vi "tpg361_set_unit.vi"() -> ()   [LabVIEW 2019]
panel:
  in  "SETTING UNIT":T1(ring)
  out "UNIT":string
  out "Overall Status":bool
  out "Acknowledgement Status":bool
  out "err_out":errorcluster
  out "tpg361_visa 2":refnum<visa-resource-name>
  in  "tpg361_b2r 2":u32
  in  "tpg361_delay 3":u32=500
  in  "tpg361_delay 2":u32=500
  in  "tpg361_b2r":u32
  in  "err_in":errorcluster
  in  "tpg361_delay":u32=500
  in  "tpg361_visa":refnum<visa-resource-name>
  # "VISA"
  # "DELAY"
  # "BYTE AT PORT"
  # "STATUS"
  # "ERROR"
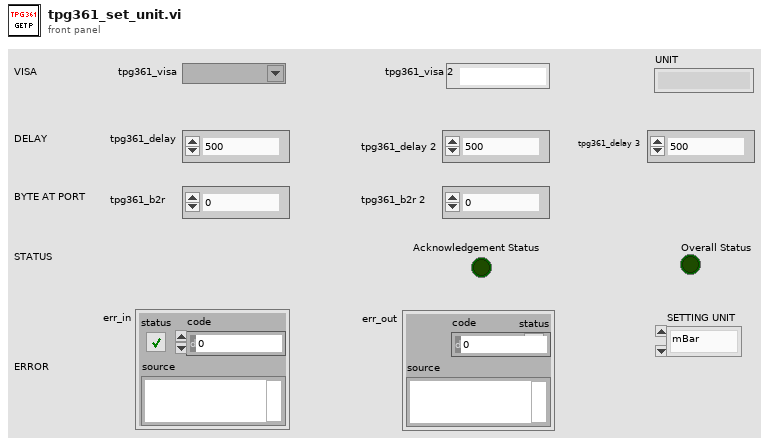
[diagram p1: front panel]
types:
  T1 = enum16{"mBar", "Torr", "Pascal", "micron", "hPascal", "Volt"}
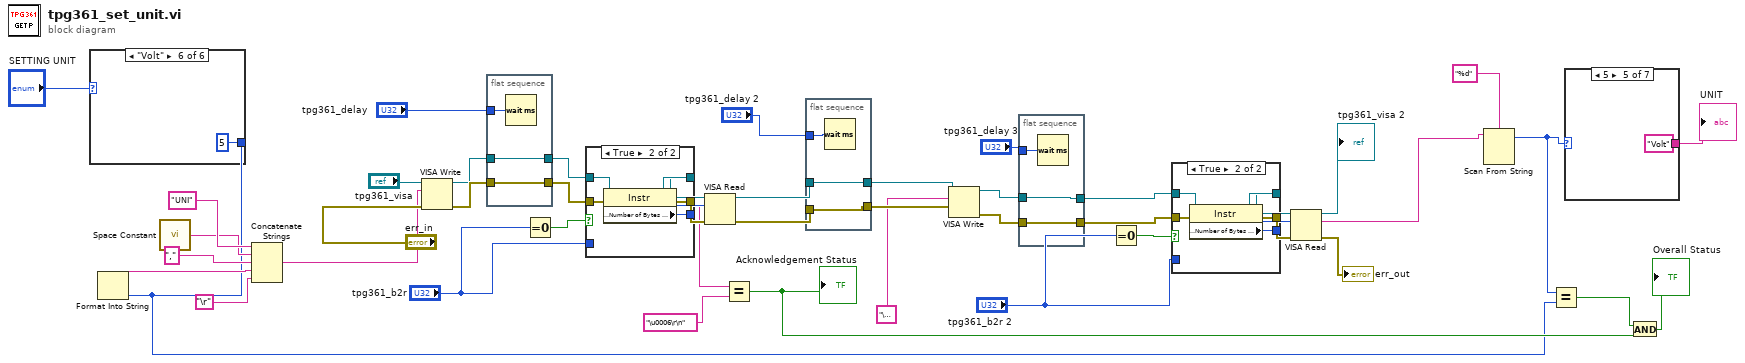
[diagram p0: block diagram]
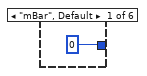
[diagram p2: hidden frame]
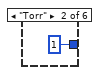
[diagram p3: hidden frame]
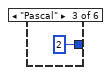
[diagram p4: hidden frame]
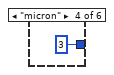
[diagram p5: hidden frame]
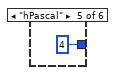
[diagram p6: hidden frame]
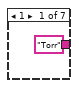
[diagram p7: hidden frame]
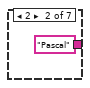
[diagram p8: hidden frame]
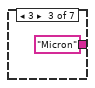
[diagram p9: hidden frame]
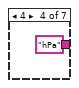
[diagram p10: hidden frame]
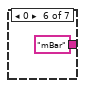
[diagram p11: hidden frame]
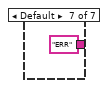
[diagram p12: hidden frame]
diagram:
  n1 = case shown="\"Volt\"" "SETTING UNIT" {
    tunnel: [0 1 2 3 4 5] -> w1
    frame "mBar", Default {
    }
    frame "Torr" {
    }
    frame "Pascal" {
    }
    frame "micron" {
    }
    frame "hPascal" {
    }
    frame "Volt" {
    }
  }
  n2 = Format Into String(w1) -> (resulting string=w6:string)  [unwired: 3 in, 1 out]
  n3 = call <vilib>:"Space Constant.vi"() -> ("String"=w8:string)
  n4 = Concatenate Strings("UNI" ("string"), w8, "," ("string"), w6, "\r") -> (w19:string)
  n5 = VISA Write(VISA resource name="tpg361_visa", write buffer=w19, error in (no error)="err_in") -> (VISA resource name out=w45:refnum<visa-resource-name>, error out=w47:errorcluster)  [unwired: 1 out]
  n6 = flat-sequence {
    tunnel: w47 -> [w55]
    tunnel: [w55] -> w46
    tunnel: w45 -> [w54]
    tunnel: [w54] -> w44
    tunnel: "tpg361_delay" -> [w56]
    frame #0 {
      n7 = Wait (ms)(milliseconds to wait=w56) -> ()  [unwired: 1 out]
    }
  }
  n8 = Equal To 0?(x="tpg361_b2r") -> (x = 0?=w40:bool)
  n9 = case shown="True" w40 {
    tunnel: w46 -> [w58 w64]
    tunnel: w44 -> [w59 w63]
    tunnel: [w59 w62] -> w38
    tunnel: [w58 w61] -> w37
    tunnel: [w57 w60] -> w36
    tunnel: "tpg361_b2r" -> [w57 _]
    frame False {
    }
    frame True {
      n10 = property class="Instr"(reference=w63, error in=w64) -> (reference out=w62:refnum<visa-resource-name>, error out=w61:errorcluster, "Serial Settings:Number of Bytes at Serial Port"=w60:u32)
    }
  }
  n11 = VISA Read(VISA resource name=w38, byte count=w36, error in (no error)=w37) -> (VISA resource name out=w35:refnum<visa-resource-name>, read buffer=w17:string, error out=w34:errorcluster)  [unwired: 1 out]
  n12 = Equal?(x=w17, y="\u0006\r\n") -> (x = y?=w13:bool)
  "Acknowledgement Status" <- w13
  n13 = flat-sequence {
    tunnel: [w65] -> w32
    tunnel: w35 -> [w67]
    tunnel: [w67] -> w33
    tunnel: "tpg361_delay 2" -> [w66]
    tunnel: w34 -> [w65]
    frame #0 {
      n14 = Wait (ms)(milliseconds to wait=w66) -> ()  [unwired: 1 out]
    }
  }
  n15 = VISA Write(VISA resource name=w33, write buffer="\u0005", error in (no error)=w32) -> (VISA resource name out=w25:refnum<visa-resource-name>, error out=w24:errorcluster)  [unwired: 1 out]
  n16 = flat-sequence {
    tunnel: [w69] -> w31
    tunnel: [w70] -> w30
    tunnel: w25 -> [w70]
    tunnel: w24 -> [w69]
    tunnel: "tpg361_delay 3" -> [w68]
    frame #0 {
      n17 = Wait (ms)(milliseconds to wait=w68) -> ()  [unwired: 1 out]
    }
  }
  n18 = Equal To 0?(x="tpg361_b2r 2") -> (x = 0?=w29:bool)
  n19 = case shown="True" w29 {
    tunnel: w31 -> [w72 w78]
    tunnel: w30 -> [w73 w77]
    tunnel: [w73 w76] -> w28
    tunnel: [w72 w75] -> w27
    tunnel: [w71 w74] -> w26
    tunnel: "tpg361_b2r 2" -> [w71 _]
    frame False {
    }
    frame True {
      n20 = property class="Instr"(reference=w77, error in=w78) -> (reference out=w76:refnum<visa-resource-name>, error out=w75:errorcluster, "Serial Settings:Number of Bytes at Serial Port"=w74:u32)
    }
  }
  n21 = VISA Read(VISA resource name=w28, byte count=w26, error in (no error)=w27) -> (VISA resource name out=→"tpg361_visa 2":refnum<visa-resource-name>, read buffer=w10:string, error out=→"err_out":errorcluster)  [unwired: 1 out]
  n22 = Scan From String(format string="%d", input string=w10) -> (output 1=w3:i32)  [unwired: 3 in, 3 out]
  n23 = Equal?(x=w3, y=w1) -> (x = y?=w2:bool)
  n24 = case shown="5" w3 {
    tunnel: ["Torr" "Pascal" "Micron" "hPa" "Volt" "mBar" "ERR"] -> w12
    frame 1 {
    }
    frame 2 {
    }
    frame 3 {
    }
    frame 4 {
    }
    frame 5 {
    }
    frame 0 {
    }
    frame Default {
    }
  }
  "UNIT" <- w12
  n25 = And(x=w2, y=w13) -> (x .and. y?=→"Overall Status":bool)
